vi "createPublisher.vi"(8 "error in (no error)":errorcluster, 11 "Boot in":refnum<class "Boot.lvclass">) -> (0 "error out":errorcluster, 2 "Publisher":refnum<class "Publisher.lvclass">, 3 "Boot out":refnum<class "Boot.lvclass">)   [LabVIEW 2016, in "Boot.lvclass"]
uses:
  Boot.lvclass
  Publisher/Publisher.lvclass
  Boot.lvclass/Boot.ctl
  Publisher/Publisher.lvclass/Publisher.ctl
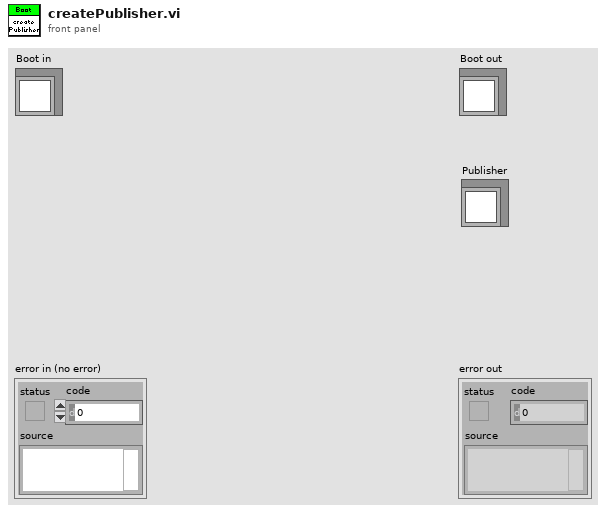
[diagram p1: front panel]
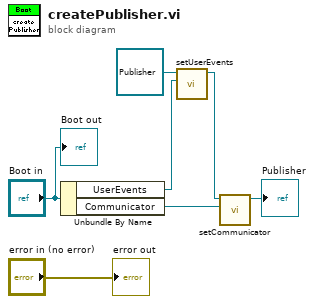
[diagram p0: block diagram]
diagram:
  n1 = Unbundle By Name("Boot in") -> ("UserEvents"=w2:refnum<class "UserEvents.lvclass">, "Communicator"=w1:refnum<class "Communicator.lvclass">)
  n2 = call "setUserEvents.vi"("UserEvents"=w2, "Publisher in"=refnum<class "Publisher.lvclass"> refnum ("Telemetry.lvclass")) -> ("Publisher out"=w5:refnum<class "Publisher.lvclass">)  [unwired: 9 in]
  n3 = call "setCommunicator.vi"("Communicator"=w1, "Publisher in"=w5) -> ("Publisher out"=→"Publisher":refnum<class "Publisher.lvclass">)  [unwired: 9 in]
  "error out" <- "error in (no error)"
  "Boot out" <- "Boot in"
